vi "Create Remote System.vi"(8 "error in (no error)":errorcluster, 9 "Size":cluster{"Width":i32, "Height":i32}, 10 "IP Address":string, 11 "System Alias":string) -> (0 "error out":errorcluster, 3 "Remote System out":refnum<class "Remote System.lvclass">)   [LabVIEW 2016, in "Remote System.lvclass"]
uses:
  Remote System.lvclass
  C:/Program Files (x86)/National Instruments/LabVIEW 2016/vi.lib/LIEF/Forms/Shape/Shape.lvclass
  C:/Program Files (x86)/National Instruments/LabVIEW 2016/vi.lib/LIEF/Forms/Rectangle/Rectangle.lvclass
  C:/Program Files (x86)/National Instruments/LabVIEW 2016/vi.lib/LIEF/Forms/Layered Shape/Layered Shape.lvclass
  <vilib>/LIEF/Forms/Shape/Shape.lvclass/Shape.ctl
  <vilib>/LIEF/Forms/Rectangle/Rectangle.lvclass/Rectangle.ctl
  <vilib>/LIEF/Forms/Layered Shape/Layered Shape.lvclass/Layered Shape.ctl
  Remote System.lvclass/Remote System.ctl
  <vilib>/LIEF/Forms/Shape/Write Movable.vi
  <vilib>/LIEF/Forms/Shape/Write Color.vi
  <vilib>/LIEF/Forms/Rectangle/Write Filled.vi
  <vilib>/LIEF/Forms/Shape/Write Selectable.vi
  <vilib>/LIEF/Forms/Layered Shape/Write Overlays.vi
  <vilib>/LIEF/Forms/Text/Text.lvclass
  <vilib>/LIEF/Forms/Shape/Shape.lvclass
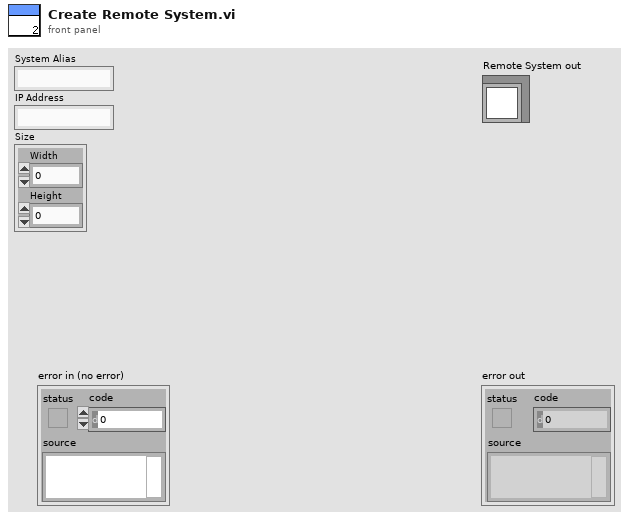
[diagram p1: front panel]
types:
  T1 = cluster{"Font Name:":string, "Size":i16, "Strikeout?":bool, "Italic?":bool, "Underline?":bool, "Outline?":bool, "Shadow?":bool, "Bold?":bool}
  T2 = enum16{"Left", "Top", "Right", "Bottom", "Centered"}
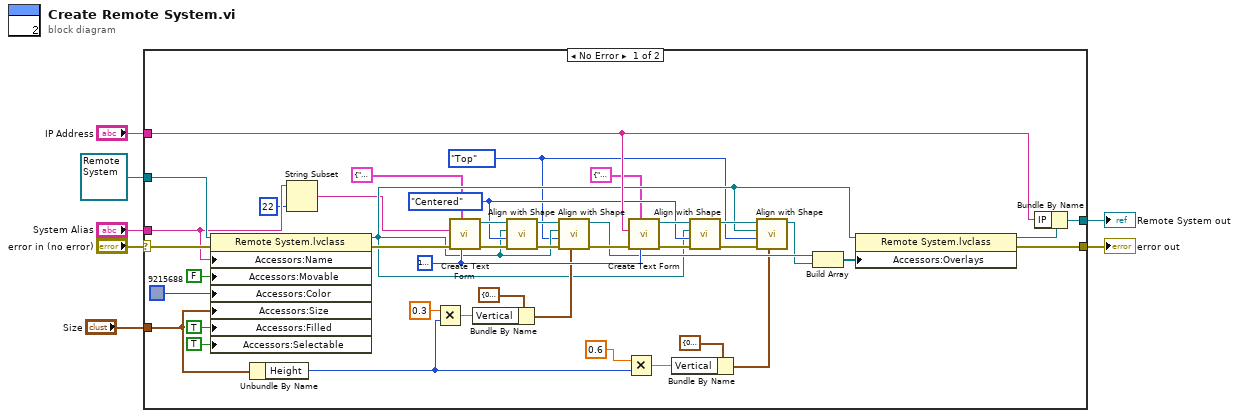
[diagram p0: block diagram]
diagram:
  n1 = case shown="No Error" "error in (no error)" {
    selector: "error in (no error)" -> [w39 w51]
    tunnel: [w41 w51] -> w6
    tunnel: [w49 w50] -> w4
    tunnel: refnum<class "Remote System.lvclass"> refnum ("Remote System in") -> [w37 w50]
    tunnel: "System Alias" -> [w10 _]
    tunnel: "IP Address" -> [w47 _]
    tunnel: "Size" -> [w32 _]
    frame No Error {
      w19 = T2."Top" ("Alignment")
      w40 = u32 16777226 ("Color")
      w33 = T2."Centered" ("Alignment")
      n2 = property class="Remote System.lvclass"(reference=w37, error in=w39, "Accessors:Name"=w10, "Accessors:Movable"=FALSE ("Movable"), "Accessors:Color"=u32 9215688, "Accessors:Size"=w32, "Accessors:Filled"=TRUE ("Filled"), "Accessors:Selectable"=TRUE ("Selectable")) -> (reference out=w20:refnum<class "Remote System.lvclass">, error out=w38:errorcluster)
      n3 = Unbundle By Name(w32) -> ("Height"=w17:i32)
      n4 = String Subset(string=w10, length (rest)=22 ("length (rest)")) -> (substring=w8:string)  [unwired: 1 in]
      n5 = Multiply(x=0.3, y=w17) -> (x*y=w25:dbl)
      n6 = call <vilib>:"Create Text Form.vi"("Color"=w40, "[user-specified font]"=T1 {"Font Name:"="Segoe UI", "Size"=18, "Strikeout?"=FALSE, "Italic?"=FALSE, "Underline?"=FALSE, "Outline?"=FALSE, "Shadow?"=FALSE, "Bold?"=TRUE}, "error in (no error)"=w38, "Text"=w8) -> ("error out"=w43:errorcluster, "New Text"=w48:refnum<class "Text.lvclass">)  [unwired: 6 in]
      n7 = Bundle By Name(cluster=cluster{"Horizontal":u32, "Vertical":u32} {"Horizontal"=0, "Vertical"=50} ("Margin"), "Vertical"=w25) -> (w24:cluster{"Horizontal":u32, "Vertical":u32})
      n8 = call <vilib>:"Align with Shape.vi"("error in (no error)"=w43, "Alignment"=w33, "Reference Shape"=w20, "Shape in"=w48) -> ("error out"=w31:errorcluster, "Shape out"=w30:refnum<class "Text.lvclass">)  [unwired: 6 in]
      n9 = call <vilib>:"Align with Shape.vi"("Margin"=w24, "error in (no error)"=w31, "Alignment"=w19, "Reference Shape"=w20, "Shape in"=w30) -> ("error out"=w29:errorcluster, "Shape out"=w28:refnum<class "Text.lvclass">)  [unwired: 5 in]
      n10 = Multiply(x=0.6, y=w17) -> (x*y=w15:dbl)
      n11 = call <vilib>:"Create Text Form.vi"("Color"=w40, "[user-specified font]"=T1 {"Font Name:"="Segoe UI", "Size"=14, "Strikeout?"=FALSE, "Italic?"=FALSE, "Underline?"=FALSE, "Outline?"=FALSE, "Shadow?"=FALSE, "Bold?"=FALSE}, "error in (no error)"=w29, "Text"=w47) -> ("error out"=w42:errorcluster, "New Text"=w46:refnum<class "Text.lvclass">)  [unwired: 6 in]
      n12 = Bundle By Name(cluster=cluster{"Horizontal":u32, "Vertical":u32} {"Horizontal"=0, "Vertical"=50} ("Margin"), "Vertical"=w15) -> (w14:cluster{"Horizontal":u32, "Vertical":u32})
      n13 = call <vilib>:"Align with Shape.vi"("error in (no error)"=w42, "Alignment"=w33, "Reference Shape"=w20, "Shape in"=w46) -> ("error out"=w22:errorcluster, "Shape out"=w23:refnum<class "Text.lvclass">)  [unwired: 6 in]
      n14 = call <vilib>:"Align with Shape.vi"("Margin"=w14, "error in (no error)"=w22, "Alignment"=w19, "Reference Shape"=w20, "Shape in"=w23) -> ("Shape out"=w21:refnum<class "Text.lvclass">)  [unwired: 5 in, 1 out]
      n15 = Build Array(w28, w21) -> (w45:refnum<class "Text.lvclass">[])
      n16 = property class="Remote System.lvclass"(reference=w20, "Accessors:Overlays"=w45) -> (reference out=w44:refnum<class "Remote System.lvclass">, error out=w41:errorcluster)  [unwired: 1 in]
      n17 = Bundle By Name(cluster=w44, "IP"=w47) -> (w49:refnum<class "Remote System.lvclass">)
    }
    frame Error {
    }
  }
  "error out" <- w6
  "Remote System out" <- w4
